vi "sendmail.vi"() -> ()   [LabVIEW 2009]
uses:
  <vilib>/Utility/SMTP/NI_SMTPEmail.lvlib
panel:
  out "source out":string
  out "message 2":string=" INSTRUCTIONS:\r\rNormal Use:  When using subVIs that incorporate the error in/error out (or error I/O) structure, place this handler where you want to inform the user of an error, typically at the end of the I/O data path, as the last action of the program.  If the error in error? is ERROR, the handler creates a message describing the error and its source.  If the type of dialog = 1 (default), the message is displayed to the user, who can only acknowedge it.  If the type = 2, the user can acknowledge the message or abort execution; aborting a program with active I/O is not recommended.  If the type = 0, no message is displayed; this is used to process the error programmatically, and the error out cluster elements are wired to individual terminals for that reason.  \r\rOther Use:\n\r\nlocal testing.  To test the error code of a subVI or function that does not have the error I/O structure, you can wire its error code and a source string to the local error code and error source inputs.  If error in error? indicates no error and error code is not equal to 0, the local code and source are substituted for the error in values, and error? is set TRUE (ERROR)."
  out "error?":bool
  in  "Send mail":bool
  in  "stop":bool
  in  "return address":string
  in  "mail server":string
  in  "recipients":string[](array[string])
  in  "message":string
  in  "subject ([No Subject])":string="[No Subject]"
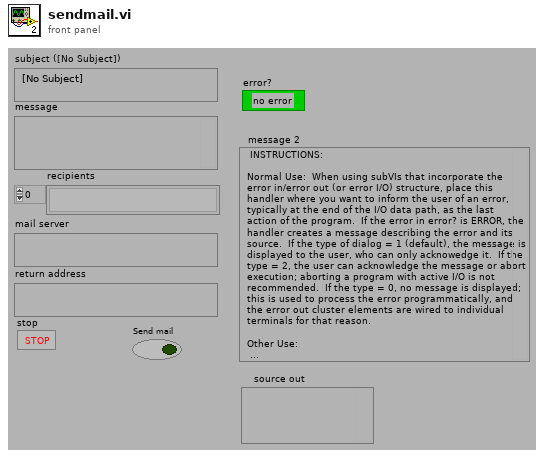
[diagram p1: front panel]
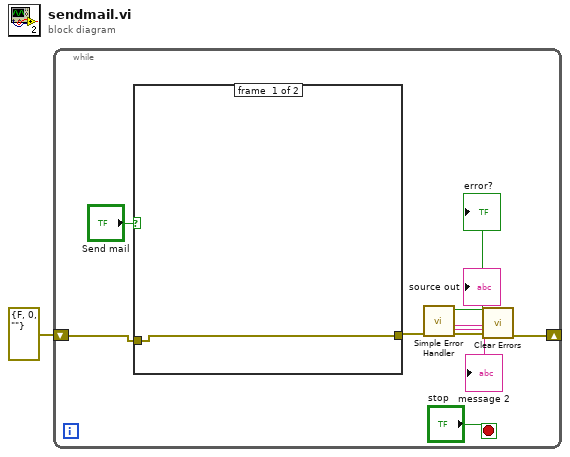
[diagram p0: block diagram]
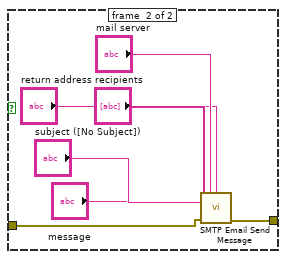
[diagram p2: hidden frame]
diagram:
  n1 = while {
    shift-right: [w5] -> _
    shift-left: errorcluster {"status"=FALSE, "code"=0, "source"=""} ("error in (no error)") -> [w8]
    stop <- "stop" stop-if-true
    n2 = case shown="True" "Send mail" {
      tunnel: w8 -> [w11 w13]
      tunnel: [w11 w12] -> w6
      frame #0 {
      }
      frame #1 {
        n3 = call <vilib>:"SMTP Email Send Message.vi"("recipients"="recipients", "mail server"="mail server", "return address"="return address", "subject ([No Subject])"="subject ([No Subject])", "message"="message", "error in (no error)"=w13) -> ("error out"=w12:errorcluster)  [unwired: 8 in, 1 out]
      }
    }
    n4 = call <vilib>:"Simple Error Handler.vi"("error in (no error)"=w6) -> ("error?"=→"error?":bool, "source out"=→"source out":string, "error out"=w7:errorcluster, "message"=→"message 2":string)  [unwired: 4 in, 1 out]
    n5 = call <vilib>:"Clear Errors.vi"("error in (no error)"=w7) -> ("error out"=w5:errorcluster)  [unwired: 6 in]
  }
